vi "hydraharp_get_nonzero_buffer.vi"(11 "buffer":u8[](array[numeric])) -> (3 "subarray":u8[](array[numeric]))   [LabVIEW 2015, in "hydraharp.lvclass"]
uses:
  hydraharp.lvclass
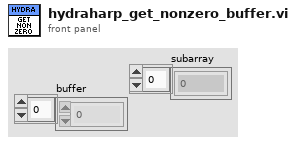
[diagram p1: front panel]
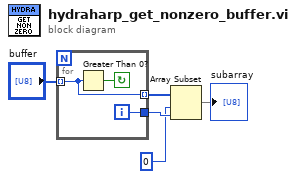
[diagram p0: block diagram]
diagram:
  n1 = for {
    tunnel: "buffer" -> [w6] mode=indexing
    tunnel: [w6] -> w3 mode=indexing
    tunnel: [w7] -> w5
    i -> [w7]
    stop <- w8 continue-if-true
    n2 = Greater Than 0?(x=w6) -> (x > 0?=w8:bool)
  }
  n3 = Array Subset(array=w3, index=0, length=w5) -> (→"subarray":u8[])
